vi "RTS Close Door.vi"(4 "Relay Number":u8=1 min=1 max=3 step=1, 6 "Station #":u8=1 min=1 max=8 step=1, 8 "Error In":errorcluster, 10 "Door Opening Controller Input":T1 {"Chamber 1-1"."Start Time" format="%<%X\n%x>T"; "Chamber 1-1"."End Time" format="%<%X\n%x>T"; "Time Count (s)" format="%.2f"}) -> (0 "Error Out":errorcluster, 2 "Door Opening Controller Output":T1 {"Chamber 1-1"."Start Time" format="%<%X\n%x>T"; "Chamber 1-1"."End Time" format="%<%X\n%x>T"; "Time Count (s)" format="%.2f"})   [LabVIEW 2016]
uses:
  Type Definitions/RTS Door Opener Indicator.ctl
  Type Definitions/RTS Door Ops Client.ctl
  Type Definitions/RTS Door Opening Schedule.ctl
  Type Definitions/RTS Door Ops Sequence.ctl
panel:
  out "8-3":dbl format="%.2f"
  out "8-2":dbl format="%.2f"
  out "8-1":dbl format="%.2f"
  out "7-3":dbl format="%.2f"
  out "7-2":dbl format="%.2f"
  out "7-1":dbl format="%.2f"
  out "6-3":dbl format="%.2f"
  out "6-2":dbl format="%.2f"
  out "6-1":dbl format="%.2f"
  out "5-3":dbl format="%.2f"
  out "5-2":dbl format="%.2f"
  out "5-1":dbl format="%.2f"
  out "4-3":dbl format="%.2f"
  out "4-2":dbl format="%.2f"
  out "4-1":dbl format="%.2f"
  out "3-3":dbl format="%.2f"
  out "3-2":dbl format="%.2f"
  out "3-1":dbl format="%.2f"
  out "2-3":dbl format="%.2f"
  out "2-2":dbl format="%.2f"
  out "2-1":dbl format="%.2f"
  out "1-3":dbl format="%.2f"
  out "1-2":dbl format="%.2f"
  out "1-1":dbl format="%.2f"
  # "Individual Timers"
  # "Chamber Conditions:"
  # "Chamber Conditions:"
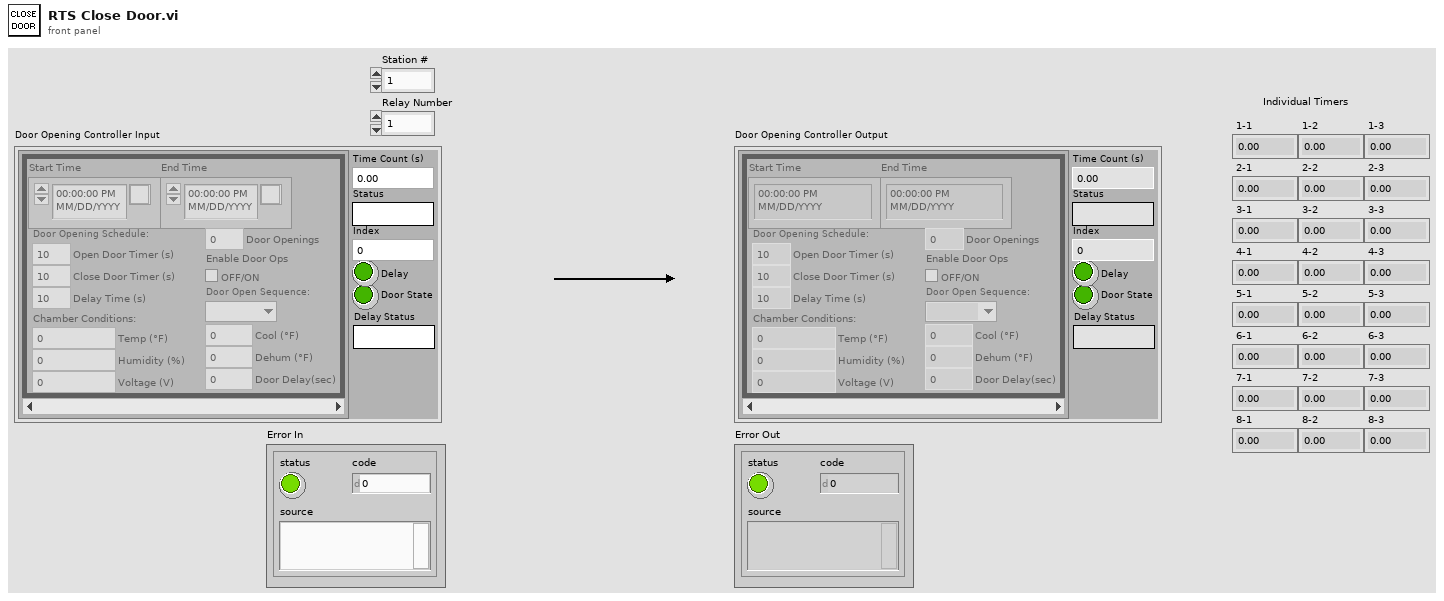
[diagram p1: front panel]
types:
  T1 = typedef "RTS Door Opener Indicator.ctl" = cluster{"Time Count (s)":dbl, "Status":string, "Door State":bool, "Delay":bool, "Chamber 1-1":T2[], "Index":i32, "Delay Status":string}
  T2 = typedef "RTS Door Ops Client.ctl" = cluster{"End Time":timestamp, "Start Time":timestamp, "Door Opening Schedule:":T3, "Enable Door Ops":bool, "Door Openings":u32, "Temp (°F)":dbl, "Humidity (%)":dbl, "Voltage (V)":dbl, "Door Open Sequence:":T4, "Door Delay(sec)":dbl, "Dehum (°F)":dbl, "Cool (°F)":dbl}
  T3 = typedef "RTS Door Opening Schedule.ctl" = cluster{"Open Door Timer (s)":dbl, "Delay Time (s)":dbl, "Close Door Timer (s)":dbl}
  T4 = typedef "RTS Door Ops Sequence.ctl" = enum16{"", "1st", "2nd", "3rd"}
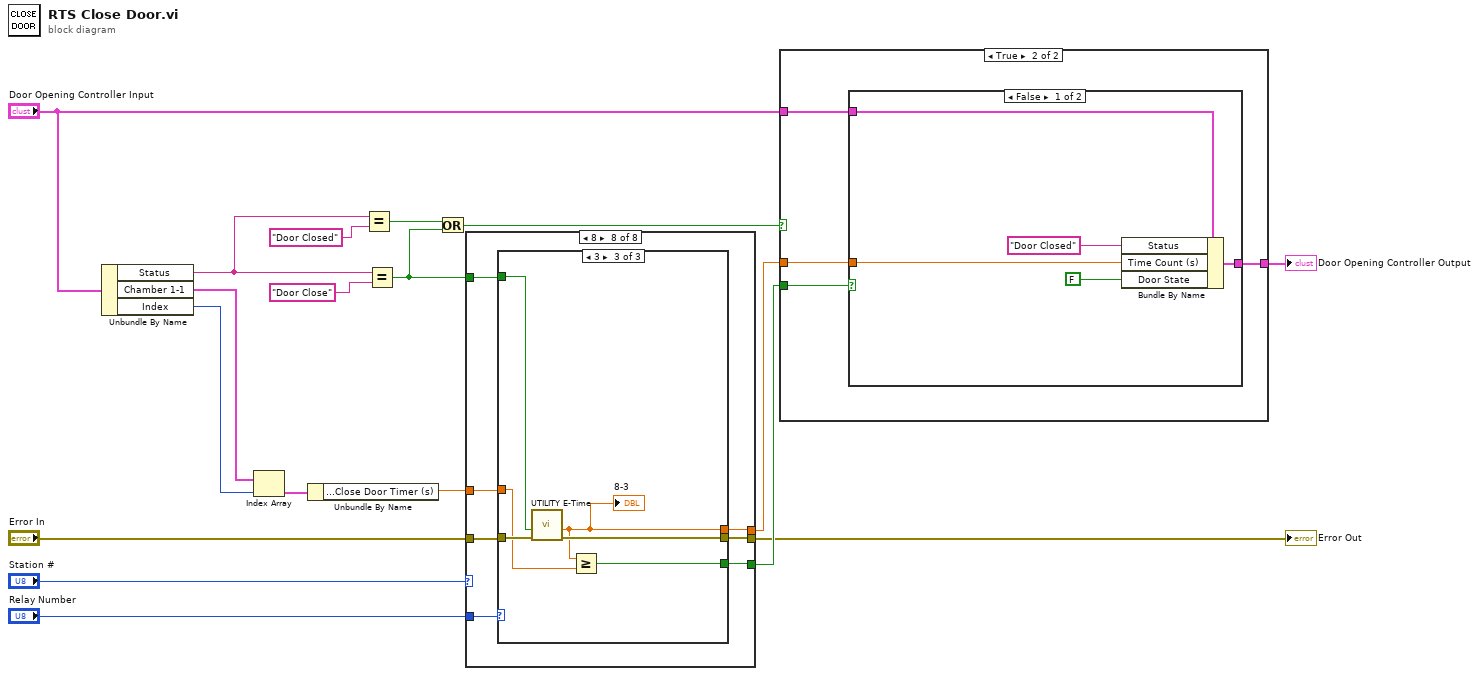
[diagram p0: block diagram]
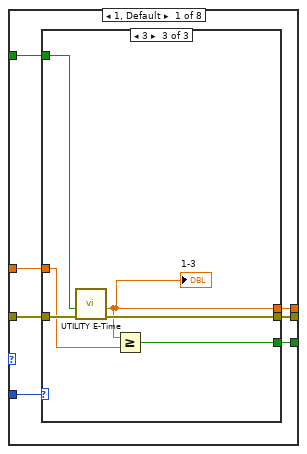
[diagram p2: hidden frame]
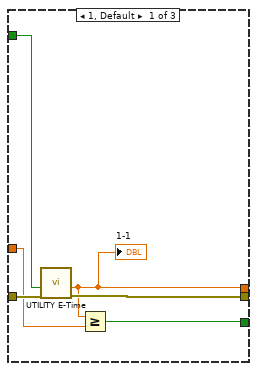
[diagram p3: hidden frame]
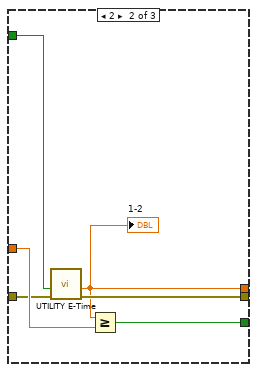
[diagram p4: hidden frame]
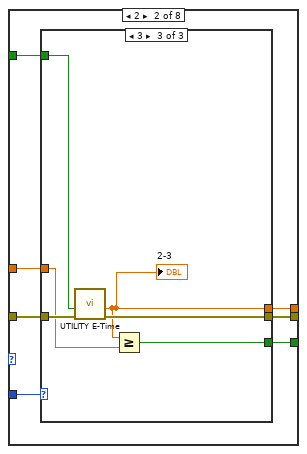
[diagram p5: hidden frame]
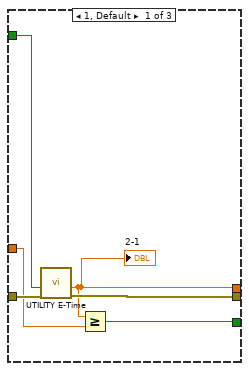
[diagram p6: hidden frame]
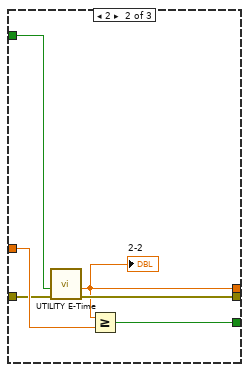
[diagram p7: hidden frame]
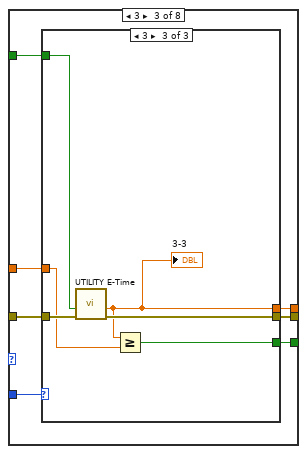
[diagram p8: hidden frame]
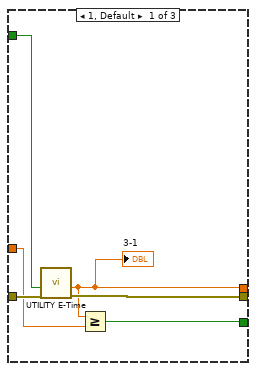
[diagram p9: hidden frame]
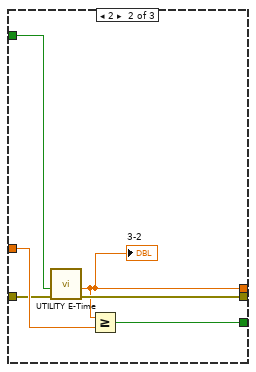
[diagram p10: hidden frame]
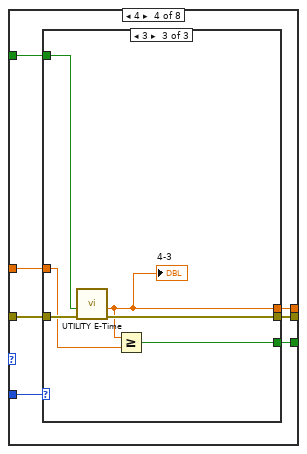
[diagram p11: hidden frame]
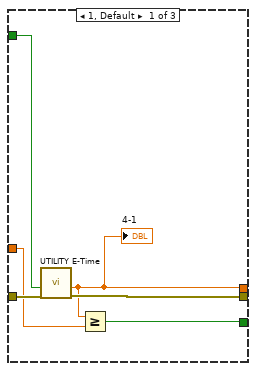
[diagram p12: hidden frame]
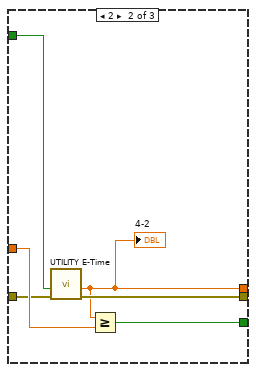
[diagram p13: hidden frame]
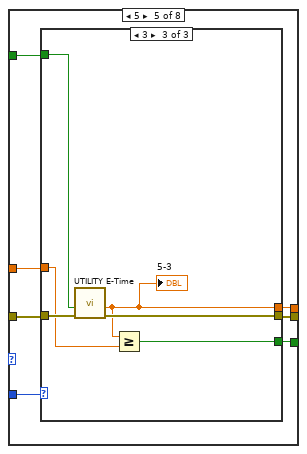
[diagram p14: hidden frame]
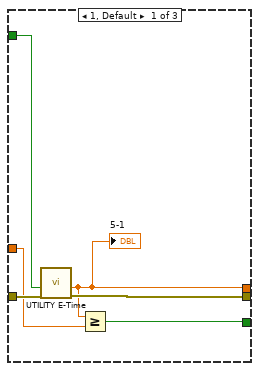
[diagram p15: hidden frame]
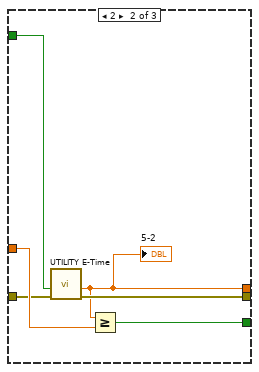
[diagram p16: hidden frame]
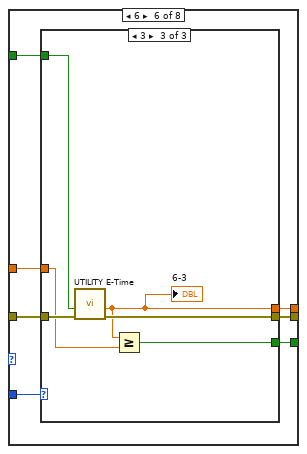
[diagram p17: hidden frame]
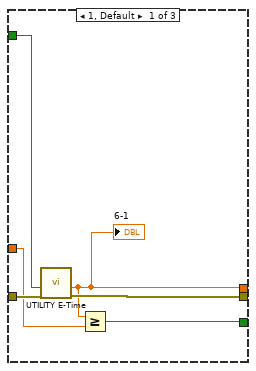
[diagram p18: hidden frame]
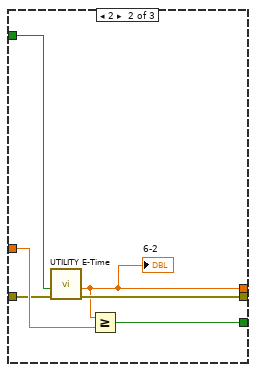
[diagram p19: hidden frame]
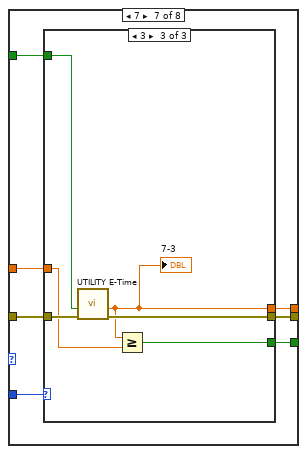
[diagram p20: hidden frame]
diagram:
  n1 = Unbundle By Name("Door Opening Controller Input") -> ("Status"=w15:string, "Chamber 1-1"=w11:T2[], "Index"=w10:i32)
  n2 = Index Array(array=w11, index=w10) -> (element=w9:T2)
  n3 = Unbundle By Name(w9) -> ("Door Opening Schedule:.Close Door Timer (s)"=w8:dbl)
  n4 = Equal?(x=w15, y="Door Closed") -> (x = y?=w13:bool)
  n5 = Equal?(x=w15, y="Door Close") -> (x = y?=w7:bool)
  n6 = Or(x=w13, y=w7) -> (x .or. y?=w12:bool)
  n7 = case shown="8" "Station #" {
    tunnel: [w25 w46 w71 w96 w121 w146 w171 w196] -> w3
    tunnel: [w24 w45 w70 w94 w119 w144 w170 w194] -> w2
    tunnel: [w23 w47 w72 w95 w120 w145 w172 w195] -> w1
    tunnel: "Error In" -> [w22 w48 w73 w98 w123 w148 w173 w198]
    tunnel: w7 -> [w21 w49 w75 w100 w125 w150 w175 w200]
    tunnel: w8 -> [w20 w44 w74 w99 w124 w149 w174 w199]
    tunnel: "Relay Number" -> [w19 w50 w69 w97 w122 w147 w169 w197]
    frame 1, Default {
      n8 = case shown="3" w19 {
        tunnel: [w29 w32 w38] -> w25
        tunnel: [w28 w35 w41] -> w24
        tunnel: [w30 w33 w42] -> w23
        tunnel: w22 -> [w31 w34 w43]
        tunnel: w21 -> [w26 w37 w39]
        tunnel: w20 -> [w27 w36 w40]
        frame 1, Default {
          n9 = call "UTILITY E-Time.vi"("error in (no error)"=w31, "Reset"=w26) -> ("error out"=w30:errorcluster, "Elapsed Time (sec)"=w29:dbl)  [unwired: 7 in, 1 out]
          "1-1" <- w29
          n10 = Greater Or Equal?(x=w29, y=w27) -> (x >= y?=w28:bool)
        }
        frame 2 {
          n11 = call "UTILITY E-Time.vi"("error in (no error)"=w34, "Reset"=w37) -> ("error out"=w33:errorcluster, "Elapsed Time (sec)"=w32:dbl)  [unwired: 7 in, 1 out]
          "1-2" <- w32
          n12 = Greater Or Equal?(x=w32, y=w36) -> (x >= y?=w35:bool)
        }
        frame 3 {
          n13 = call "UTILITY E-Time.vi"("error in (no error)"=w43, "Reset"=w39) -> ("error out"=w42:errorcluster, "Elapsed Time (sec)"=w38:dbl)  [unwired: 7 in, 1 out]
          "1-3" <- w38
          n14 = Greater Or Equal?(x=w38, y=w40) -> (x >= y?=w41:bool)
        }
      }
    }
    frame 2 {
      n15 = case shown="3" w50 {
        tunnel: [w51 w57 w63] -> w46
        tunnel: [w54 w60 w66] -> w45
        tunnel: [w55 w58 w67] -> w47
        tunnel: w48 -> [w56 w59 w68]
        tunnel: w49 -> [w52 w62 w64]
        tunnel: w44 -> [w53 w61 w65]
        frame 1, Default {
          n16 = call "UTILITY E-Time.vi"("error in (no error)"=w56, "Reset"=w52) -> ("error out"=w55:errorcluster, "Elapsed Time (sec)"=w51:dbl)  [unwired: 7 in, 1 out]
          "2-1" <- w51
          n17 = Greater Or Equal?(x=w51, y=w53) -> (x >= y?=w54:bool)
        }
        frame 2 {
          n18 = call "UTILITY E-Time.vi"("error in (no error)"=w59, "Reset"=w62) -> ("error out"=w58:errorcluster, "Elapsed Time (sec)"=w57:dbl)  [unwired: 7 in, 1 out]
          "2-2" <- w57
          n19 = Greater Or Equal?(x=w57, y=w61) -> (x >= y?=w60:bool)
        }
        frame 3 {
          n20 = call "UTILITY E-Time.vi"("error in (no error)"=w68, "Reset"=w64) -> ("error out"=w67:errorcluster, "Elapsed Time (sec)"=w63:dbl)  [unwired: 7 in, 1 out]
          "2-3" <- w63
          n21 = Greater Or Equal?(x=w63, y=w65) -> (x >= y?=w66:bool)
        }
      }
    }
    frame 3 {
      n22 = case shown="3" w69 {
        tunnel: [w76 w82 w88] -> w71
        tunnel: [w79 w85 w91] -> w70
        tunnel: [w80 w83 w92] -> w72
        tunnel: w73 -> [w81 w84 w93]
        tunnel: w75 -> [w77 w87 w89]
        tunnel: w74 -> [w78 w86 w90]
        frame 1, Default {
          n23 = call "UTILITY E-Time.vi"("error in (no error)"=w81, "Reset"=w77) -> ("error out"=w80:errorcluster, "Elapsed Time (sec)"=w76:dbl)  [unwired: 7 in, 1 out]
          "3-1" <- w76
          n24 = Greater Or Equal?(x=w76, y=w78) -> (x >= y?=w79:bool)
        }
        frame 2 {
          n25 = call "UTILITY E-Time.vi"("error in (no error)"=w84, "Reset"=w87) -> ("error out"=w83:errorcluster, "Elapsed Time (sec)"=w82:dbl)  [unwired: 7 in, 1 out]
          "3-2" <- w82
          n26 = Greater Or Equal?(x=w82, y=w86) -> (x >= y?=w85:bool)
        }
        frame 3 {
          n27 = call "UTILITY E-Time.vi"("error in (no error)"=w93, "Reset"=w89) -> ("error out"=w92:errorcluster, "Elapsed Time (sec)"=w88:dbl)  [unwired: 7 in, 1 out]
          "3-3" <- w88
          n28 = Greater Or Equal?(x=w88, y=w90) -> (x >= y?=w91:bool)
        }
      }
    }
    frame 4 {
      n29 = case shown="3" w97 {
        tunnel: [w101 w107 w113] -> w96
        tunnel: [w104 w110 w116] -> w94
        tunnel: [w105 w108 w117] -> w95
        tunnel: w98 -> [w106 w109 w118]
        tunnel: w100 -> [w102 w112 w114]
        tunnel: w99 -> [w103 w111 w115]
        frame 1, Default {
          n30 = call "UTILITY E-Time.vi"("error in (no error)"=w106, "Reset"=w102) -> ("error out"=w105:errorcluster, "Elapsed Time (sec)"=w101:dbl)  [unwired: 7 in, 1 out]
          "4-1" <- w101
          n31 = Greater Or Equal?(x=w101, y=w103) -> (x >= y?=w104:bool)
        }
        frame 2 {
          n32 = call "UTILITY E-Time.vi"("error in (no error)"=w109, "Reset"=w112) -> ("error out"=w108:errorcluster, "Elapsed Time (sec)"=w107:dbl)  [unwired: 7 in, 1 out]
          "4-2" <- w107
          n33 = Greater Or Equal?(x=w107, y=w111) -> (x >= y?=w110:bool)
        }
        frame 3 {
          n34 = call "UTILITY E-Time.vi"("error in (no error)"=w118, "Reset"=w114) -> ("error out"=w117:errorcluster, "Elapsed Time (sec)"=w113:dbl)  [unwired: 7 in, 1 out]
          "4-3" <- w113
          n35 = Greater Or Equal?(x=w113, y=w115) -> (x >= y?=w116:bool)
        }
      }
    }
    frame 5 {
      n36 = case shown="3" w122 {
        tunnel: [w126 w132 w138] -> w121
        tunnel: [w129 w135 w141] -> w119
        tunnel: [w130 w133 w142] -> w120
        tunnel: w123 -> [w131 w134 w143]
        tunnel: w125 -> [w127 w137 w139]
        tunnel: w124 -> [w128 w136 w140]
        frame 1, Default {
          n37 = call "UTILITY E-Time.vi"("error in (no error)"=w131, "Reset"=w127) -> ("error out"=w130:errorcluster, "Elapsed Time (sec)"=w126:dbl)  [unwired: 7 in, 1 out]
          "5-1" <- w126
          n38 = Greater Or Equal?(x=w126, y=w128) -> (x >= y?=w129:bool)
        }
        frame 2 {
          n39 = call "UTILITY E-Time.vi"("error in (no error)"=w134, "Reset"=w137) -> ("error out"=w133:errorcluster, "Elapsed Time (sec)"=w132:dbl)  [unwired: 7 in, 1 out]
          "5-2" <- w132
          n40 = Greater Or Equal?(x=w132, y=w136) -> (x >= y?=w135:bool)
        }
        frame 3 {
          n41 = call "UTILITY E-Time.vi"("error in (no error)"=w143, "Reset"=w139) -> ("error out"=w142:errorcluster, "Elapsed Time (sec)"=w138:dbl)  [unwired: 7 in, 1 out]
          "5-3" <- w138
          n42 = Greater Or Equal?(x=w138, y=w140) -> (x >= y?=w141:bool)
        }
      }
    }
    frame 6 {
      n43 = case shown="3" w147 {
        tunnel: [w151 w157 w163] -> w146
        tunnel: [w154 w160 w166] -> w144
        tunnel: [w155 w158 w167] -> w145
        tunnel: w148 -> [w156 w159 w168]
        tunnel: w150 -> [w152 w162 w164]
        tunnel: w149 -> [w153 w161 w165]
        frame 1, Default {
          n44 = call "UTILITY E-Time.vi"("error in (no error)"=w156, "Reset"=w152) -> ("error out"=w155:errorcluster, "Elapsed Time (sec)"=w151:dbl)  [unwired: 7 in, 1 out]
          "6-1" <- w151
          n45 = Greater Or Equal?(x=w151, y=w153) -> (x >= y?=w154:bool)
        }
        frame 2 {
          n46 = call "UTILITY E-Time.vi"("error in (no error)"=w159, "Reset"=w162) -> ("error out"=w158:errorcluster, "Elapsed Time (sec)"=w157:dbl)  [unwired: 7 in, 1 out]
          "6-2" <- w157
          n47 = Greater Or Equal?(x=w157, y=w161) -> (x >= y?=w160:bool)
        }
        frame 3 {
          n48 = call "UTILITY E-Time.vi"("error in (no error)"=w168, "Reset"=w164) -> ("error out"=w167:errorcluster, "Elapsed Time (sec)"=w163:dbl)  [unwired: 7 in, 1 out]
          "6-3" <- w163
          n49 = Greater Or Equal?(x=w163, y=w165) -> (x >= y?=w166:bool)
        }
      }
    }
    frame 7 {
      n50 = case shown="3" w169 {
        tunnel: [w176 w182 w188] -> w171
        tunnel: [w179 w185 w191] -> w170
        tunnel: [w180 w183 w192] -> w172
        tunnel: w173 -> [w181 w184 w193]
        tunnel: w175 -> [w177 w187 w189]
        tunnel: w174 -> [w178 w186 w190]
        frame 1, Default {
          n51 = call "UTILITY E-Time.vi"("error in (no error)"=w181, "Reset"=w177) -> ("error out"=w180:errorcluster, "Elapsed Time (sec)"=w176:dbl)  [unwired: 7 in, 1 out]
          "7-1" <- w176
          n52 = Greater Or Equal?(x=w176, y=w178) -> (x >= y?=w179:bool)
        }
        frame 2 {
          n53 = call "UTILITY E-Time.vi"("error in (no error)"=w184, "Reset"=w187) -> ("error out"=w183:errorcluster, "Elapsed Time (sec)"=w182:dbl)  [unwired: 7 in, 1 out]
          "7-2" <- w182
          n54 = Greater Or Equal?(x=w182, y=w186) -> (x >= y?=w185:bool)
        }
        frame 3 {
          n55 = call "UTILITY E-Time.vi"("error in (no error)"=w193, "Reset"=w189) -> ("error out"=w192:errorcluster, "Elapsed Time (sec)"=w188:dbl)  [unwired: 7 in, 1 out]
          "7-3" <- w188
          n56 = Greater Or Equal?(x=w188, y=w190) -> (x >= y?=w191:bool)
        }
      }
    }
    frame 8 {
      n57 = case shown="3" w197 {
        tunnel: [w201 w207 w213] -> w196
        tunnel: [w204 w210 w216] -> w194
        tunnel: [w205 w208 w217] -> w195
        tunnel: w198 -> [w206 w209 w218]
        tunnel: w200 -> [w202 w212 w214]
        tunnel: w199 -> [w203 w211 w215]
        frame 1, Default {
          n58 = call "UTILITY E-Time.vi"("error in (no error)"=w206, "Reset"=w202) -> ("error out"=w205:errorcluster, "Elapsed Time (sec)"=w201:dbl)  [unwired: 7 in, 1 out]
          "8-1" <- w201
          n59 = Greater Or Equal?(x=w201, y=w203) -> (x >= y?=w204:bool)
        }
        frame 2 {
          n60 = call "UTILITY E-Time.vi"("error in (no error)"=w209, "Reset"=w212) -> ("error out"=w208:errorcluster, "Elapsed Time (sec)"=w207:dbl)  [unwired: 7 in, 1 out]
          "8-2" <- w207
          n61 = Greater Or Equal?(x=w207, y=w211) -> (x >= y?=w210:bool)
        }
        frame 3 {
          n62 = call "UTILITY E-Time.vi"("error in (no error)"=w218, "Reset"=w214) -> ("error out"=w217:errorcluster, "Elapsed Time (sec)"=w213:dbl)  [unwired: 7 in, 1 out]
          "8-3" <- w213
          n63 = Greater Or Equal?(x=w213, y=w215) -> (x >= y?=w216:bool)
        }
      }
    }
  }
  "Error Out" <- w1
  n64 = case shown="True" w12 {
    tunnel: [w219 w223] -> w18
    tunnel: "Door Opening Controller Input" -> [w219 w222]
    tunnel: w3 -> [_ w221]
    tunnel: w2 -> [_ w220]
    frame False {
    }
    frame True {
      n65 = case shown="False" w220 {
        tunnel: w222 -> [w228 w232]
        tunnel: [w227 w231] -> w223
        tunnel: w221 -> [w226 _]
        frame False {
          n66 = Bundle By Name(cluster=w228, "Status"="Door Closed" ("y"), "Time Count (s)"=w226, "Door State"=FALSE ("Open Door")) -> (w227:T1)
        }
        frame True {
          n67 = Bundle By Name(cluster=w232, "Status"="", "Delay"=TRUE) -> (w231:T1)
        }
      }
    }
  }
  "Door Opening Controller Output" <- w18
